vi "FPGA Control of one WS2812 string.vi"(9 "FPGA DO line":refnum<k21>, 10 "Wire ID":u8, 11 "FIFO In":refnum<k21>="Dispersal 4") -> ()   [LabVIEW 2025]
uses:
  <vilib>/Platform/TimedLoop/XDataNode/timing_clust.ctl
  <vilib>/Platform/TimedLoop/XDataNode/nitl_modes.ctl
  <vilib>/Platform/TimedLoop/XDataNode/wakeup.ctl
  <vilib>/rvi/Emulation/niFpgaGetClockAttributes.vi
  <vilib>/rvi/Emulation/niFpgaSctlEmulationGetInTimedLoop.vi
  <vilib>/rvi/Emulation/niFpgaEmulationReportErrorSimple.vi
  <vilib>/rvi/DataTransferAndStorage/Container/Common/niFpgaContainerGetUniqueNameForEmu.vi
  <vilib>/rvi/DataTransferAndStorage/Container/Common/niFpgaContainerSetEmuInfo.vi
  <vilib>/rvi/eio/common/nirviEmuReportErrorAndStop.vi
  <vilib>/rvi/DataTransferAndStorage/Container/Common/niFpgaContainerExecOnDevCompGetState.vi
  <vilib>/rvi/Emulation/niFpgaEmulationIsFPGAContextNoSignature.vi
  <vilib>/rvi/errors/niFpgaSetErrorForExecOnDevCompSimple.vi
  <vilib>/rvi/FIFO/Fifo_Resource/nirvififoEmulationSetSize.vi
  <vilib>/rvi/FIFO/Fifo_Resource/nirviFifoEmulationQueueMgr.vi
  <instcachedir>/0/nirviFifoEmulationQueueMgr_E5CAEC123FF24DC58D834DCA3CDAA9B5.lvgen/nirviFifoEmulationQueueMgr_E5CAEC123FF24DC58D834DCA3CDAA9B5_002.vi
  <vilib>/rvi/FIFO/Fifo_Resource/nirvififoEmulationDetermineInputValidOut.vi
  <vilib>/rvi/FIFO/Fifo_Resource/nirvififoEmulationCreateLock.vi
  <vilib>/rvi/Emulation/niFpgaProcessEmulError.vi
  <vilib>/rvi/FIFO/Fifo_Resource/nirvififoEmulationObtainLock.vi
  <vilib>/rvi/FIFO/Fifo_Resource/nirvififoEmulationReleaseLock.vi
  <vilib>/rvi/occurrence/nirviWaitOnOccurrenceBase.vi
  <vilib>/rvi/errors/nirviReportUnexpectedCaseInternalError.vi
  <vilib>/rvi/errors/nirviReportUnexpectedCaseInternalError (U32).vi
  <vilib>/Utility/error.llb/Clear Errors.vi
  <vilib>/eio/utilities/niEioResolveVilibRelativePath.vi
  <vilib>/rvi/interface/RandomDataEmulation/niFpgaRandomDataHandleErrors.vi
  <instcachedir>/0/nirviFifoEmulationQueueMgr_E5CAEC123FF24DC58D834DCA3CDAA9B5.lvgen/nirviFifoEmulationQueueMgr_E5CAEC123FF24DC58D834DCA3CDAA9B5_001.vi
  <vilib>/rvi/Emulation/niFpgaCriticalErrorInLSC.vi
  <vilib>/rvi/eio/common/nirviEmuTemplateMethod_errors.vi
  <vilib>/Platform/TimedLoop/XDataNode/XDataNode.xnode
  <vilib>/rvi/LocalResourceManager/LocalResourceManager.xnode
  <vilib>/rvi/DataTransferAndStorage/Container/XNode/niFpgaContainer.xnode
  <vilib>/rvi/FIFO/Fifo_Resource/niFpgaFifoEmulationRefIn.vi
  <vilib>/eio/EIONode/EIONode.xnode
  <vilib>/Platform/TimedLoop/XDataNode/XDNodeRunTimeDep.lvlib
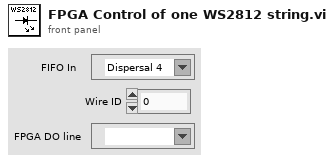
[diagram p1: front panel]
types:
  T1 = typedef "XDNodeRunTimeDep.lvlib/timing_clust.ctl" = cluster{"Expected End [f-1]":u64, "Actual End [f-1]":u64, "Finished Late? [f-1]":bool, "Expected End [i-1]":u64, "Actual End [i-1]":u64, "Finished Late? [i-1]":bool, "Expected Start [i]":u64, "Actual Start [i]":u64, "Expected Start [f]":u64, "Actual Start [f]":u64, "Source Name":string, "Structure Name":string, "Period":i64, "Deadline":i64, "Offset":i64, "Start":i64, "Priority":i32, "Timeout":i32, "Mode":T2, "Wakeup Reason":T3, "Error":errorcluster, "Source Type":string, "Secondary Source Type":string, "Global End Time":u64, "Global Start Time":u64, "Frame Duration":u64, "Iteration Duration":u64, "Assigned CPU":i32, "I/O Scan Engine Mode":u32}
  T2 = typedef "XDNodeRunTimeDep.lvlib/nitl_modes.ctl" = enum32{"No Change", "Process missed periods, maintain original phase", "Discard missed periods, maintain original phase", "Process missed periods, ignore original phase", "Discard missed periods, ignore original phase"}
  T3 = typedef "XDNodeRunTimeDep.lvlib/wakeup.ctl" = enum32{"Normal", "Aborted", "Asynchronous wakeup", "Timing source error", "Timed loop error", "Timeout"}
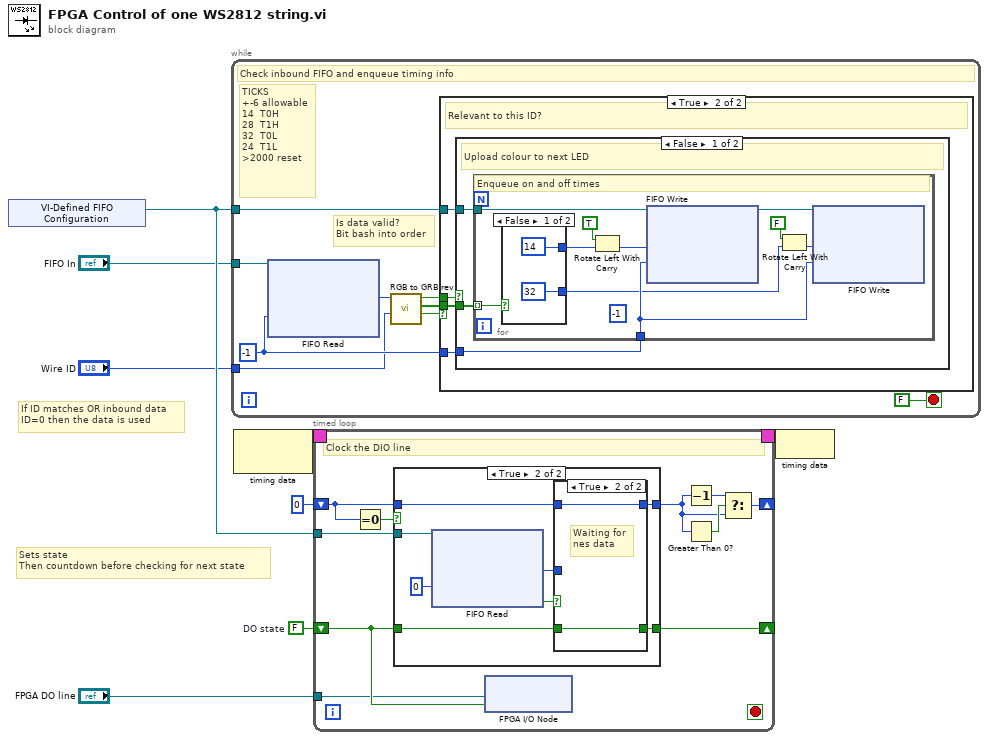
[diagram p0: block diagram]
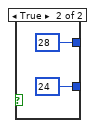
[diagram p3: hidden frame]
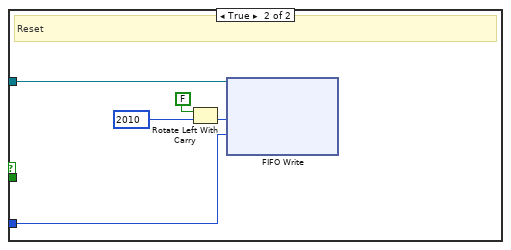
[diagram p4: hidden frame]
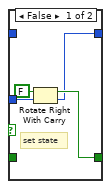
[diagram p6: hidden frame]
diagram:
  w5 = FALSE  # DO state
  # "If ID matches OR inbound data\nID=0 then the data is used"
  # "Sets state \nThen countdown before checking for next state"
  n1 = xnode "VI-Defined FIFO Configuration"() -> ("FIFO Out"=w3:refnum<k21>)
  n2 = while {
    tunnel: w3 -> [w17]
    tunnel: "FIFO In" -> [w11]
    tunnel: "Wire ID" -> [w10]
    stop <- FALSE stop-if-true
    w15 = -1 ("Timeout")
    # "Is data valid?\nBit bash into order"
    # "TICKS\n+-6 allowable\n14  T0H\n28  T1H\n32  T0L\n24  T1L\n>2000 reset"
    # "Check inbound FIFO and enqueue timing info"
    n3 = xnode ("FIFO Read")("Timeout"=w15, "FIFO In"=w11) -> ("Element"=w13:u32)  [unwired: 2 out]
    n4 = call "RGB to GRB rev.vi"("ID"=w10, "Element"=w13) -> ("Valid"=w9:bool, "Array"=w12:bool[], "Reset"=w14:bool)  [unwired: 7 in]
    n5 = case shown="True" w9 {
      tunnel: w17 -> [_ w21]
      tunnel: w15 -> [_ w20]
      tunnel: w14 -> [_ w19]
      tunnel: w12 -> [_ w18]
      frame False {
      }
      frame True {
        # "Relevant to this ID?"
        n6 = case shown="False" w19 {
          tunnel: w21 -> [w24 w43]
          tunnel: w20 -> [w23 w42]
          tunnel: w18 -> [w22 _]
          frame False {
            # "Upload colour to next LED"
            n7 = for {
              tunnel: w24 -> [w34]
              tunnel: w22 -> [w32] mode=indexing
              tunnel: w23 -> [w31]
              (unwired) -1 ("Timeout")
              # "Enqueue on and off times"
              n8 = case shown="False" w32 {
                tunnel: [u16 14 u16 28] -> w30
                tunnel: [u16 32 u16 24] -> w27
                frame False {
                }
                frame True {
                }
              }
              n9 = Rotate Left With Carry(2:w30, 3:TRUE ("carry")) -> (0:w29:u16)  [unwired: 1 out]
              n10 = xnode ("FIFO Write")("Element"=w29, "Timeout"=w31, "FIFO In"=w34) -> ("FIFO Out"=w33:refnum<k21>)  [unwired: 1 out]
              n11 = Rotate Left With Carry(2:w27, 3:FALSE ("carry")) -> (0:w25:u16)  [unwired: 1 out]
              n12 = xnode ("FIFO Write")("Element"=w25, "Timeout"=w31, "FIFO In"=w33) -> ()  [unwired: 2 out]
            }
          }
          frame True {
            # "Reset"
            n13 = Rotate Left With Carry(2:u16 2010, 3:FALSE ("carry")) -> (0:w40:u16)  [unwired: 1 out]
            n14 = xnode ("FIFO Write")("Element"=w40, "Timeout"=w42, "FIFO In"=w43) -> ()  [unwired: 2 out]
          }
        }
      }
    }
  }
  n15 = node-c288() -> (w8:T1)  [unwired: 1 in]
  n16 = timed-loop {
    timing: w8 -> [_]
    timing-out: [_] -> w7
    shift-right: [w51] -> _
    shift-left: u16 0 -> [w47]
    tunnel: w3 -> [w50]
    shift-right: [w46] -> _
    shift-left: w5 -> [w45]
    tunnel: "FPGA DO line" -> [w44]
    stop <- _ stop-if-true
    # "Clock the DIO line"
    n17 = Equal To 0?(x=w47) -> (x = 0?=w49:bool)
    n18 = case shown="True" w49 {
      tunnel: w50 -> [_ w63]
      tunnel: [w55 w59] -> w48
      tunnel: w47 -> [w55 w57]
      tunnel: [w54 w61] -> w46
      tunnel: w45 -> [w54 w56]
      frame False {
      }
      frame True {
        n19 = xnode ("FIFO Read")("Timeout"=0, "FIFO In"=w63) -> ("Element"=w60:u16, "Timed Out?"=w58:bool)  [unwired: 1 out]
        n20 = case shown="True" w58 {
          tunnel: [w67 w68] -> w61
          tunnel: w60 -> [w66 _]
          tunnel: [w65 w69] -> w59
          tunnel: w57 -> [_ w69]
          tunnel: w56 -> [_ w68]
          frame False {
            # "set state"
            n21 = Rotate Right With Carry(2:w66, 3:FALSE ("carry")) -> (0:w65:u16, 1:w67:bool)
          }
          frame True {
            # "Waiting for\nnes data"
          }
        }
      }
    }
    n22 = xnode "FPGA I/O Node"("I/O Item"=w45, "FPGA I/O In"=w44) -> ()  [unwired: 1 out]
    n23 = Decrement(x=w48) -> (x-1=w52:u16)
    n24 = Greater Than 0?(x=w48) -> (x > 0?=w53:bool)
    n25 = Select(t=w52, s=w53, f=w48) -> (s? t:f=w51:u16)
  }
  n26 = node-c288(w7) -> ()
